vi "Example Callback - Quaternion Callback.vi"(4 "Quaternion":refnum<user-event>, 5 "Event Data":T1, 6 "Control Ref":refnum<k24>, 7 "Event Common Data":T2) -> ()   [LabVIEW 2010]
uses:
  C:/tf/play/labview/Tinkerforge.dll
  Tinkerforge.dll
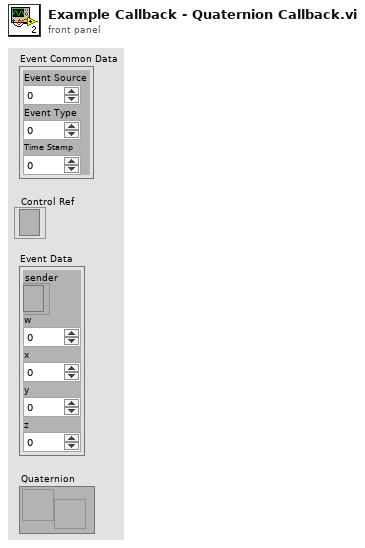
[diagram p1: front panel]
types:
  T1 = cluster{"sender":refnum<k24>, "w":i16, "x":i16, "y":i16, "z":i16}
  T2 = cluster{"Event Source":i32, "Event Type":u32, "Time Stamp":u32}
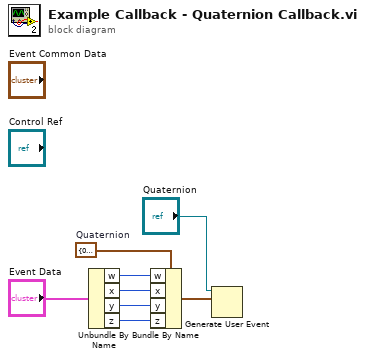
[diagram p0: block diagram]
diagram:
  w4 = cluster{"w":i16, "x":i16, "y":i16, "z":i16} {"w"=0, "x"=0, "y"=0, "z"=0}  # Quaternion
  n1 = Unbundle By Name("Event Data") -> ("w"=w8:i16, "x"=w7:i16, "y"=w6:i16, "z"=w5:i16)
  n2 = Bundle By Name(cluster=w4, "w"=w8, "x"=w7, "y"=w6, "z"=w5) -> (w3:cluster{"w":i16, "x":i16, "y":i16, "z":i16})
  n3 = Generate User Event(user event="Quaternion", event data cluster=w3) -> ()  [unwired: 1 in, 2 out]
